vi "cm_Calculate Levels.vi"(8 "error in (no error)":errorcluster, 9 "Linear View":bool, 10 "Channel Info":T3(array[cluster]), 11 "Data In":T2) -> (0 "error out":errorcluster, 2 "Channel Status":T1[](array[typedef]) {"Current Level" scale=0.0..1.0; "Peak Level" scale=0.0..1.0}, 3 "Channel Info":T3(array[cluster]))   [LabVIEW 2012, in "Channel Monitor.xctl"]
uses:
  Channel Monitor.xctl
  TypeDef/cm_Channel Indicator.ctl
  cm_Channel Monitor Data.ctl
panel:
  in  "Channel Status 2":T1 {"Current Level" scale=0.0..1.0; "Peak Level" scale=0.0..1.0}
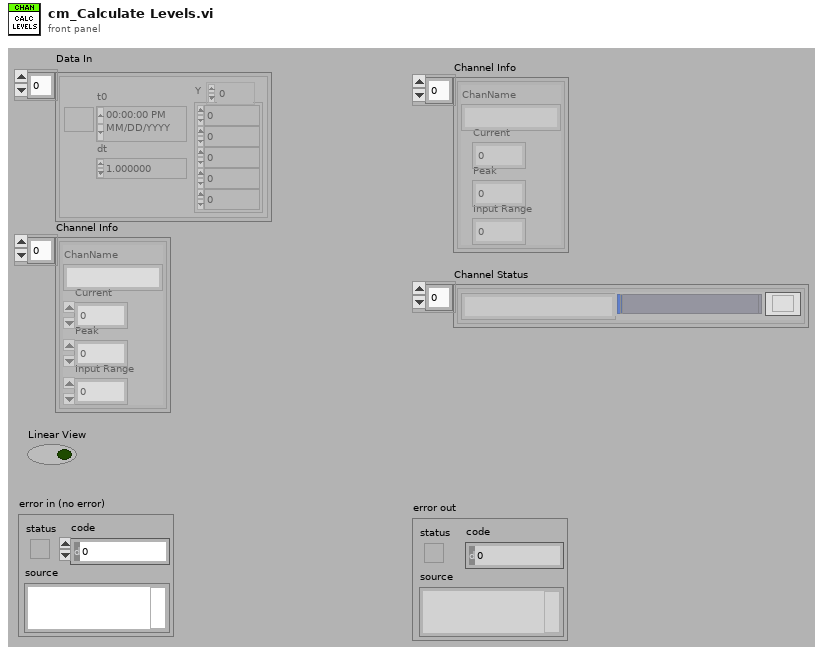
[diagram p1: front panel]
types:
  T1 = typedef "Channel Monitor.xctl/cm_Channel Indicator.ctl" = cluster{"Channel Name":string, "TimeDomain":bool, "Peak Level":dbl, "Current Level":dbl}
  T2 = typedef "Channel Monitor.xctl/cm_Channel Monitor Data.ctl" = waveform(dbl)[]
  T3 = cluster{"ChanName":string, "Current":dbl, "Peak":dbl, "Input Range":dbl}[]
  T4 = cluster{"ChanName":string, "Current":dbl, "Peak":dbl, "Input Range":dbl}
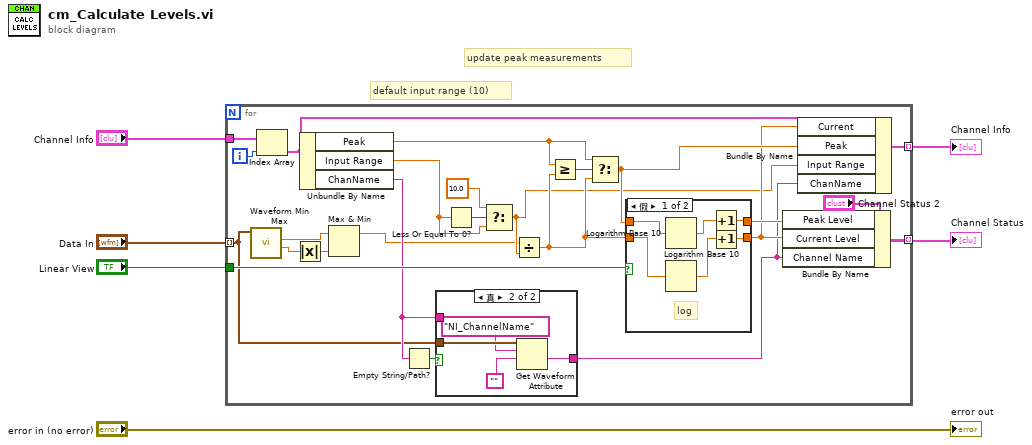
[diagram p0: block diagram]
diagram:
  # "default input range (10)"
  # "update peak measurements"
  n1 = for {
    tunnel: "Data In" -> [w13] mode=indexing
    tunnel: [w31] -> w2 mode=indexing
    tunnel: "Channel Info" -> [w27]
    tunnel: [w30] -> w5 mode=indexing
    tunnel: "Linear View" -> [w26]
    i -> [w23]
    n2 = call <vilib>:"Waveform Min Max.vi"("waveform in"=w13) -> ("Y min"=w11:dbl, "Y max"=w12:dbl)  [unwired: 5 in, 4 out]
    n3 = Index Array(array=w27, index=w23) -> (element=w20:T4)
    n4 = Absolute Value(x=w11) -> (abs(x)=w10:dbl)
    n5 = Unbundle By Name(w20) -> ("Peak"=w28:dbl, "Input Range"=w19:dbl, "ChanName"=w17:string)
    n6 = Max & Min(x=w12, y=w10) -> (max(x,y)=w9:dbl)  [unwired: 1 out]
    n7 = Empty String/Path?(string/path=w17) -> (empty?=w18:bool)
    n8 = case shown="真" w18 {
      tunnel: w13 -> [_ w36]
      tunnel: [w32 w35] -> w7
      tunnel: w17 -> [w32 _]
      frame False {
      }
      frame True {
        n9 = Get Waveform Attribute(5:"", 6:"NI_ChannelName" ("name"), 7:w36) -> (1:w35:string)  [unwired: 1 in, 3 out]
      }
    }
    n10 = Less Or Equal To 0?(x=w19) -> (x <= 0?=w22:bool)
    n11 = Select(t=10.0 ("y"), s=w22, f=w19) -> (s? t:f=w14:dbl)
    n12 = Divide(x=w9, y=w14) -> (x/y=w24:dbl)
    n13 = Greater Or Equal?(x=w28, y=w24) -> (x >= y?=w29:bool)
    n14 = Select(t=w28, s=w29, f=w24) -> (s? t:f=w16:dbl)
    n15 = case shown="假" w26 {
      tunnel: w16 -> [w42 w44]
      tunnel: w24 -> [w41 w43]
      tunnel: [w39 w44] -> w25
      tunnel: [w38 w43] -> w15
      frame False {
        # "log"
        n16 = Logarithm Base 10(1:w42) -> (0:w40:dbl)
        n17 = Logarithm Base 10(1:w41) -> (0:w37:dbl)
        n18 = Increment(x=w40) -> (x+1=w39:dbl)
        n19 = Increment(x=w37) -> (x+1=w38:dbl)
      }
      frame True {
      }
    }
    n20 = Bundle By Name(cluster="Channel Status 2", "Peak Level"=w25, "Current Level"=w15, "Channel Name"=w7) -> (w31:T1)
    n21 = Bundle By Name(cluster=w20, "Current"=w15, "Peak"=w16, "Input Range"=w14, "ChanName"=w7) -> (w30:T4)
  }
  "Channel Info" <- w5
  "Channel Status" <- w2
  "error out" <- "error in (no error)"
